vi "Msg.vi"(7 "jettl in":refnum<class "jettl.lvclass">, 11 "Iterate Msg Strategy in":refnum<class "Iterate Msg Strategy.lvclass">) -> (5 "jettl out":refnum<class "jettl.lvclass">)   [LabVIEW 2021, in "Hello World Event.lvlib" / "Iterate Msg Strategy.lvlib" / "Iterate Msg Strategy.lvclass"]
uses:
  Iterate Msg Strategy.lvclass
  <vilib>/Nathan Davis/jettl/jettl/jettl/jettl.lvclass
  Iterate/Iterate.lvclass
  Iterate Msg Strategy.lvclass/Iterate Msg Strategy.ctl
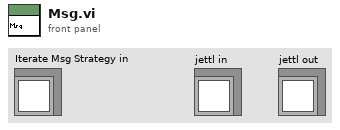
[diagram p1: front panel]
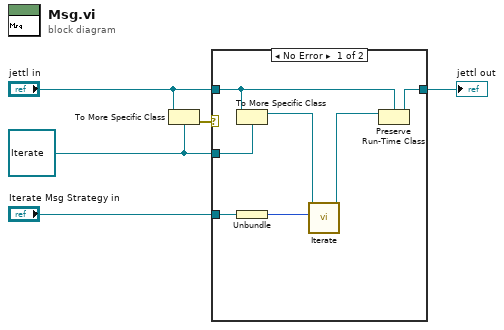
[diagram p0: block diagram]
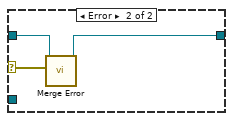
[diagram p2: hidden frame]
diagram:
  w2 = refnum<class "Iterate.lvclass"> refnum ("jettl Msg Template")
  n1 = To More Specific Class(target class=w2, reference="jettl in") -> (error out=w5:errorcluster)  [unwired: 1 in, 1 out]
  n2 = case shown="No Error" w5 {
    selector: w5 -> [_ w14]
    tunnel: [w10 w13] -> w3
    tunnel: "jettl in" -> [w11 w15]
    tunnel: w2 -> [w12 _]
    tunnel: "Iterate Msg Strategy in" -> [w7 _]
    frame No Error {
      n3 = To More Specific Class(target class=w12, reference=w11) -> (specific class reference=w9:refnum<class "Iterate.lvclass">)  [unwired: 1 in, 1 out]
      n4 = Unbundle "Unbundle"(w7) -> (w6:i32)
      n5 = call-dynamic "Iterate.vi"("Iterate"=w6, "Iterate in"=w9) -> ("Iterate out"=w8:refnum<class "Iterate.lvclass">)  [unwired: 9 in]
      n6 = Preserve Run-Time Class(object in=w8, 2:w11) -> (object out=w10:refnum<class "jettl.lvclass">)  [unwired: 1 in, 1 out]
    }
    frame Error {
      n7 = call-dynamic "Merge Error.vi"("Error"=w14, "Merge Error in"=w15) -> ("Merge Error out"=w13:refnum<class "jettl.lvclass">)  [unwired: 9 in]
    }
  }
  "jettl out" <- w3
